vi "CSGaussmeter.RelDisplay.vi"(5 "Extrem_Value":T1, 7 "Boolean":bool, 11 "error in (no error)":errorcluster) -> (6 "Answer":string, 8 "Boolean 2":bool, 15 "error out":errorcluster)   [LabVIEW 2014, in "CSGaussmeter.lvlib"]
uses:
  CSGaussmeter.lvlib
  instr.lib/FH_55/TypeDef/Value_String.ctl
  instr.lib/FH_55/FH 55.lvlib
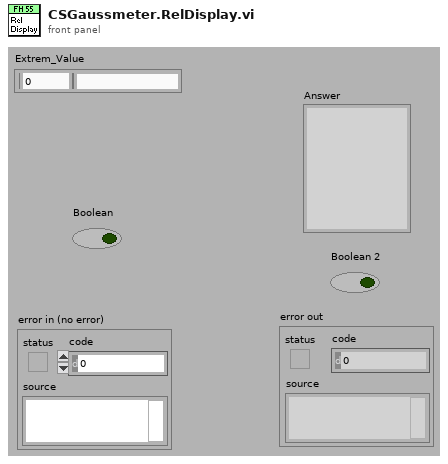
[diagram p1: front panel]
types:
  T1 = typedef "FH 55.lvlib/Value_String.ctl" = cluster{"Numeric":dbl, "String":string}
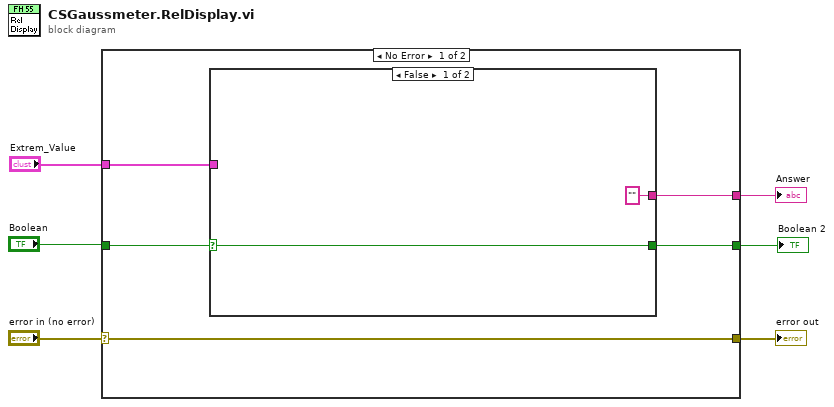
[diagram p0: block diagram]
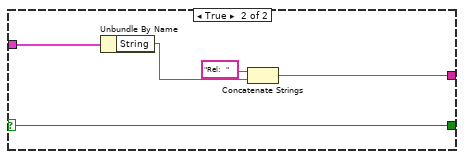
[diagram p2: hidden frame]
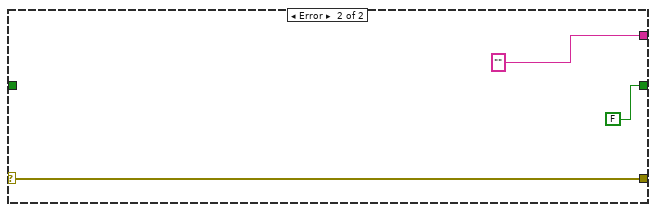
[diagram p3: hidden frame]
diagram:
  n1 = case shown="No Error" "error in (no error)" {
    selector: "error in (no error)" -> [w8 w21]
    tunnel: [w10 "" ("Answer")] -> w6
    tunnel: "Boolean" -> [w11 _]
    tunnel: [w8 w21] -> w4
    tunnel: [w9 FALSE] -> w2
    tunnel: "Extrem_Value" -> [w7 _]
    frame No Error {
      n2 = case shown="False" w11 {
        selector: w11 -> [w12 w16]
        tunnel: ["" w17] -> w10
        tunnel: [w12 w16] -> w9
        tunnel: w7 -> [_ w14]
        frame False {
        }
        frame True {
          n3 = Unbundle By Name(w14) -> ("String"=w15:string)
          n4 = Concatenate Strings("Rel:   " ("string"), w15) -> (w17:string)
        }
      }
    }
    frame Error {
    }
  }
  "Answer" <- w6
  "error out" <- w4
  "Boolean 2" <- w2
